vi "Flattened String to String.vi"(9 "Offset":u32, 10 "Flattened String":string) -> (1 "Offset After String":u32, 2 "String":string)   [LabVIEW 2013, in "OpenConvert.lvlib"]
uses:
  OpenConvert.lvlib
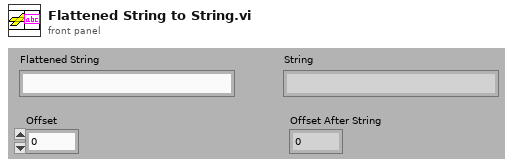
[diagram p1: front panel]
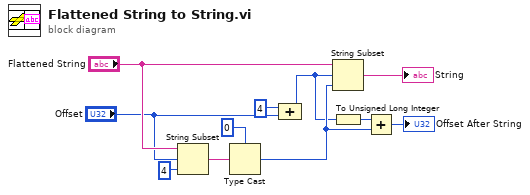
[diagram p0: block diagram]
diagram:
  n1 = String Subset(string="Flattened String", offset (0)="Offset", length (rest)=4 ("offset (0)")) -> (substring=w10:string)
  n2 = Type Cast(type=u32 0, x=w10) -> (*(type *) &x=w3:u32)
  n3 = Compound Arithmetic op=ADD(u32 4 ("offset (0)"), "Offset") -> (w2:u32)
  n4 = String Subset(string="Flattened String", offset (0)=w2, length (rest)=w3) -> (substring=→"String":string)
  n5 = To Unsigned Long Integer(number=w2) -> (unsigned 32bit integer=w5:u32)
  n6 = Add(x=w5, y=w3) -> (x+y=→"Offset After String":u32)
